vi "SwerveDriveFuse.vi"(0 "Strafe Joystick Axes":cluster{"X":dbl, "Y":dbl}, 1 "Face Joystick Axes":cluster{"X":dbl, "Y":dbl}, 2 "Trigger Axes":cluster{"Left":dbl, "Right":dbl}, 3 "Face PID Gains":T8={"proportional gain (Kc)"=0.275, "integral time (Ti, min)"=0.0, "derivative time (Td, min)"=0.006} {"derivative time (Td, min)" format="%.3f"; "integral time (Ti, min)" format="%.3f"; "proportional gain (Kc)" format="%.3f"}, 4 "Angle (degrees; 0 = right)":dbl, 5 "error in (no error)":errorcluster, 6 "Strafe Multiplier":dbl, 8 "Rotation Multiplier":dbl, 10 "Max Wheel Speed":dbl) -> (16 "Speed Chart":cluster{dbl, "Encoder Velocity":dbl}[](graph), 19 "error out":errorcluster)   [LabVIEW 2015, in "Team900SwerveDrive.lvlib"]
uses:
  Team900SwerveDrive.lvlib
  <vilib>/Rock Robotics/WPI/MotorControl/WPI_MotorControlDeviceRef.ctl
  <vilib>/Rock Robotics/WPI/MotorControl/WPI_MotorControlType.ctl
  <vilib>/Rock Robotics/SystemInterfaces/DIO/FPGA_DIOPWMChannel.ctl
  <vilib>/Rock Robotics/WPI/PWM/WPI_PWMDeadband.ctl
  <vilib>/Rock Robotics/WPI/CAN/Jaguar/SubVIs/WPI_CANJaguar_ControlMode.ctl
  <vilib>/Rock Robotics/WPI/CAN/TalonSRX/WPI_CANTalonSRX_APIControlMode.ctl
  SwerveDriveRotate.vi
  SwerveDriveFace.vi
panel:
  in  "Steering Motor Refs":T1[](array[typedef])
  in  "Speed Motor Refs":T1[](array[typedef])
  # "Run this to drive the robot in teleop; expects values\nfor max speed (in units of encoder velocity), each \nof the multipliers (between 0 and 1), robot angle, and\ninput devices (strafe joystick axes drive the robot \naround the field; face joystick axes give the robot a \ntarget angle based on the angle of the joystick; \ntriggers rotate the robot  constantly (right: clockwise,\nleft: counterclockwise). Expects the Y axes of the \njoysticks to be -1 for full up, 1 for full down as this is \nhow it is on the logitech controllers.\n\nThought: change the inputs to be more abstract \nrather than expecting a particular input device\n(see WPI's arcade and tank drive)"
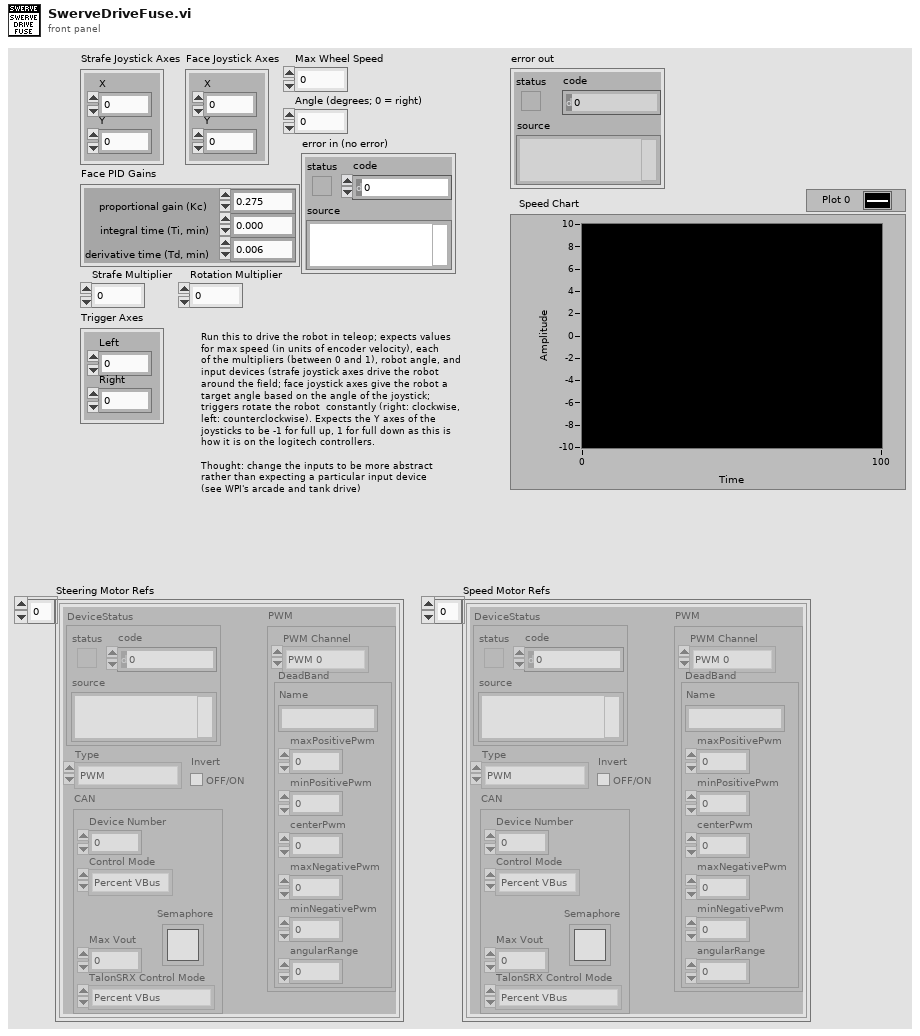
[diagram p1: front panel]
types:
  T1 = typedef "WPI_MotorControlDeviceRef.ctl" = cluster{"DeviceStatus":errorcluster, "Type":T2, "PWM":cluster{"PWM Channel":T3, "DeadBand":T4}, "CAN":cluster{"Device Number":u8, "Control Mode":T5, "Semaphore":T6, "Max Vout":dbl, "TalonSRX Control Mode":T7}, "Invert":bool}
  T2 = typedef "WPI_MotorControlType.ctl" = enum16{"PWM", "CAN", "CANTalonSRX"}
  T3 = typedef "FPGA_DIOPWMChannel.ctl" = enum8{"PWM 0", "PWM 1", "PWM 2", "PWM 3", "PWM 4", "PWM 5", "PWM 6", "PWM 7", "PWM 8", "PWM 9", "PWM MXP 0", "PWM MXP 1", "PWM MXP 2", "PWM MXP 3", "PWM MXP 4", "PWM MXP 5", "PWM MXP 6", "PWM MXP 7", "PWM MXP 8", "PWM MXP 9", "Invalid"}
  T4 = typedef "WPI_PWMDeadband.ctl" = cluster{"Name":string, "maxPositivePwm":i32, "minPositivePwm":i32, "centerPwm":i32, "maxNegativePwm":i32, "minNegativePwm":i32, "angularRange":u16}
  T5 = typedef "WPI_CANJaguar_ControlMode.ctl" = enum8{"Percent VBus", "Current", "Speed", "Position", "Voltage"}
  T6 = typedef "Semaphore RefNum" = refnum<k1>
  T7 = typedef "WPI_CANTalonSRX_APIControlMode.ctl" = enum8{"Percent VBus", "Speed", "Position", "Slave", "Unchanged / Invalid", "Voltage Compensation", "Current", "Motion Profile"}
  T8 = cluster{"proportional gain (Kc)":dbl, "integral time (Ti, min)":dbl, "derivative time (Td, min)":dbl}
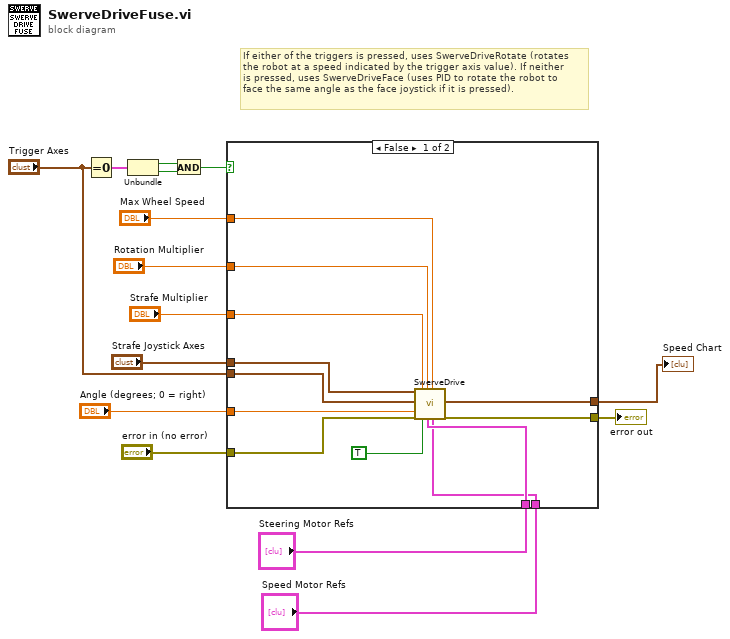
[diagram p0: block diagram]
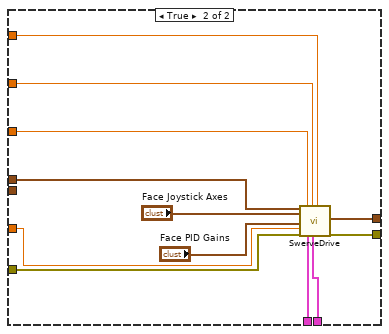
[diagram p2: hidden frame]
diagram:
  # "If either of the triggers is pressed, uses SwerveDriveRotate (rotates\nthe robot at a speed indicated by the trigger axis value). If neither\nis pressed, uses SwerveDriveFace (uses PID to rotate the robot to\nface the same angle as the face joystick if it is pressed)."
  n1 = Equal To 0?(x="Trigger Axes") -> (x = 0?=w8:cluster{"Left":bool, "Right":bool})
  n2 = Unbundle(w8) -> ("Left"=w7:bool, "Right"=w6:bool)
  n3 = And(x=w7, y=w6) -> (x .and. y?=w5:bool)
  n4 = case shown="False" w5 {
    tunnel: "Strafe Joystick Axes" -> [w23 w39]
    tunnel: "Strafe Multiplier" -> [w21 w36]
    tunnel: "Rotation Multiplier" -> [w20 w35]
    tunnel: "Max Wheel Speed" -> [w19 w34]
    tunnel: "Angle (degrees; 0 = right)" -> [w22 w33]
    tunnel: "error in (no error)" -> [w26 w32]
    tunnel: [w27 w31] -> w9
    tunnel: "Trigger Axes" -> [w24 _]
    tunnel: [w18 w30] -> w3
    tunnel: "Steering Motor Refs" -> [w17 w29]
    tunnel: "Speed Motor Refs" -> [w16 w28]
    frame False {
      n5 = call-poly "SwerveDrive.vi"("Strafe Joystick Axes"=w23, "Trigger Axes"=w24, "Angle (degrees; 0 = right)"=w22, "error in (no error)"=w26, "Strafe Multiplier"=w21, "FieldCentric? (T)"=TRUE, "Rotation Multiplier"=w20, "Steering Motor Refs"=w17, "Max Wheel Speed"=w19, "Speed Motor Refs"=w16) -> ("Speed Chart"=w18:cluster{dbl, "Encoder Velocity":dbl}[], "error out"=w27:errorcluster)  [unwired: 7 in, 1 out]
    }
    frame True {
      n6 = call-poly "SwerveDrive.vi"("Strafe Joystick Axes"=w39, "Face Joystick Axes"="Face Joystick Axes", "Face PID Gains"="Face PID Gains", "Angle (degrees; 0 = right)"=w33, "error in (no error)"=w32, "Strafe Multiplier"=w36, "Steering Motor Refs"=w29, "Rotation Multiplier"=w35, "Speed Motor Refs"=w28, "Max Wheel Speed"=w34) -> ("Speed Chart"=w30:cluster{dbl, "Encoder Velocity":dbl}[], "error out"=w31:errorcluster)  [unwired: 8 in]
    }
  }
  "error out" <- w9
  "Speed Chart" <- w3
